vi "Initialize.vi"(8 "error in":errorcluster, 11 "Plugin in":refnum<class "Tone Measurements.lvclass">) -> (0 "error out":errorcluster, 3 "Plugin out":refnum<class "Tone Measurements.lvclass">)   [LabVIEW 2025, in "Tone Measurements.lvlib" / "Tone Measurements.lvclass"]
uses:
  Tone Measurements.lvclass
  C:/Program Files/National Instruments/LabVIEW 2025/vi.lib/FlexLogger/SDK/PluginSDK.lvlibp/PEFClasses/SDK/Plugin/Plugin.lvclass
  <vilib>/FlexLogger/SDK/PluginSDK.lvlibp/PEFClasses/SDK/Producer Channel/Producer Channel.lvclass
  C:/Program Files/National Instruments/LabVIEW 2025/vi.lib/FlexLogger/SDK/PluginSDK.lvlibp/PEFClasses/SDK/Channel/Channel.lvclass
  <vilib>/FlexLogger/SDK/PluginSDK.lvlibp/PEFClasses/SDK/Plugin/ParameterAccess/Write Single Channel.vi
  <vilib>/FlexLogger/SDK/PluginSDK.lvlibp/PEFClasses/SDK/Plugin/ParameterAccess/Write DBL.vi
  <vilib>/FlexLogger/SDK/PluginSDK.lvlibp/PEFClasses/SDK/Plugin/ParameterAccess/Write I32.vi
  <vilib>/FlexLogger/SDK/PluginSDK.lvlibp/PEFClasses/SDK/Producer Channel/Create Producer Channel_v2.vi
  <vilib>/FlexLogger/SDK/PluginSDK.lvlibp/PEFClasses/SDK/Plugin/Plugin.lvclass
  C:/Program Files/National Instruments/LabVIEW 2025/vi.lib/FlexLogger/SDK/PluginSDK.lvlibp/PEFClasses/SDK/Processing Element/Processing Element.lvclass
  C:/dev/dsb/niflexlogger-plugins/PDK plugins/Tone Measurements/Tone Measurements.lvclass
  <vilib>/FlexLogger/SDK/PluginSDK.lvlibp
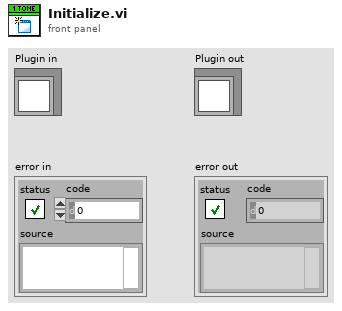
[diagram p1: front panel]
types:
  T1 = cluster{"Unique Channel Identifier":string, "Long Name":string, "Unit":string}[]
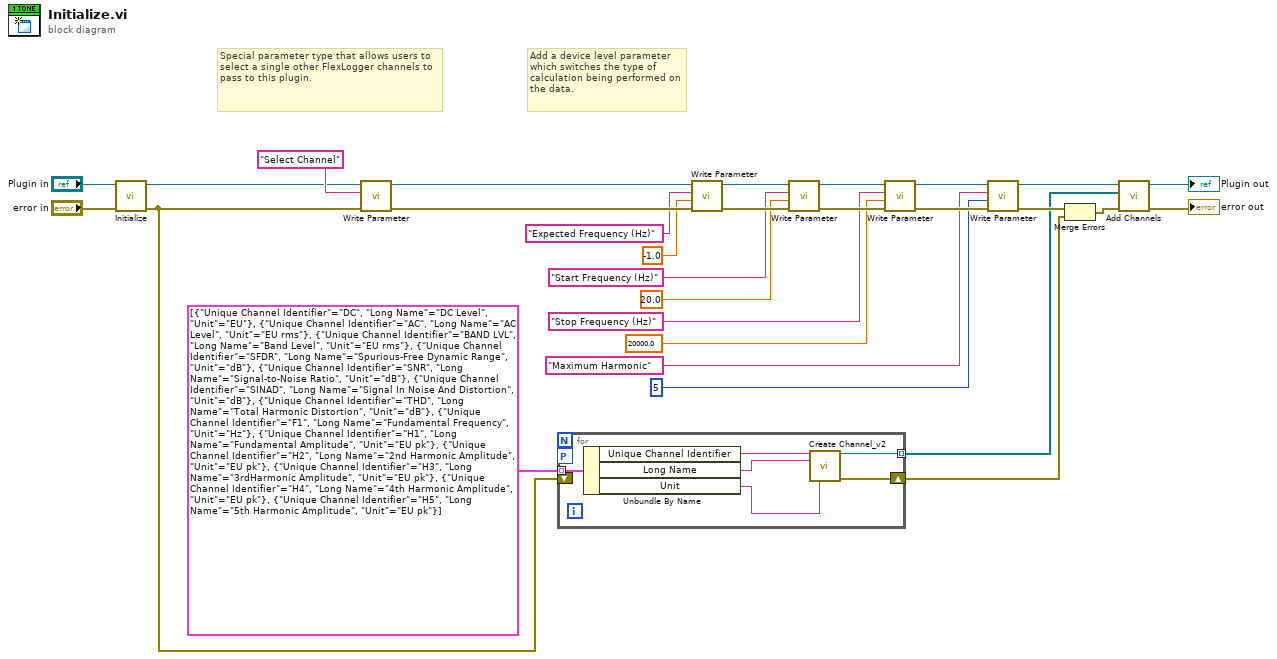
[diagram p0: block diagram]
diagram:
  # "Add a device level parameter which switches the type of calculation being performed on the data."
  # "Special parameter type that allows users to select a single other FlexLogger channels to pass to this plugin."
  n1 = call-parent "Initialize.vi"("error in (no error)"="error in", "Plugin in"="Plugin in") -> ("error out"=w2:errorcluster, "Plugin out"=w21:refnum<class "Tone Measurements.lvclass">)  [unwired: 8 in]
  n2 = call-poly <vilib>:"Write Parameter.vi"("error in (no error)"=w2, "Name (Unique Channel Identifier)"="Select Channel" ("Name"), "Plugin in"=w21) -> ("error out"=w23:errorcluster, "Plugin out"=w24:refnum<class "Tone Measurements.lvclass">)  [unwired: 7 in]
  n3 = for {
    tunnel: T1 [{"Unique Channel Identifier"="DC", "Long Name"="DC Level", "Unit"="EU"}, {"Unique Channel Identifier"="AC", "Long Name"="AC Level", "Unit"="EU rms"}, {"Unique Channel Identifier"="BAND LVL", "Long Name"="Band Level", "Unit"="EU rms"}, {"Unique Channel Identifier"="SFDR", "Long Name"="Spurious-Free Dynamic Range", "Unit"="dB"}, {"Unique Channel Identifier"="SNR", "Long Name"="Signal-to-Noise Ratio", "Unit"="dB"}, {"Unique Channel Identifier"="SINAD", "Long Name"="Signal In Noise And Distortion", "Unit"="dB"}, {"Unique Channel Identifier"="THD", "Long Name"="Total Harmonic Distortion", "Unit"="dB"}, {"Unique Channel Identifier"="F1", "Long Name"="Fundamental Frequency", "Unit"="Hz"}, {"Unique Channel Identifier"="H1", "Long Name"="Fundamental Amplitude", "Unit"="EU pk"}, {"Unique Channel Identifier"="H2", "Long Name"="2nd Harmonic Amplitude", "Unit"="EU pk"}, {"Unique Channel Identifier"="H3", "Long Name"="3rdHarmonic Amplitude", "Unit"="EU pk"}, {"Unique Channel Identifier"="H4", "Long Name"="4th Harmonic Amplitude", "Unit"="EU pk"}, {"Unique Channel Identifier"="H5", "Long Name"="5th Harmonic Amplitude", "Unit"="EU pk"}] -> [w35] mode=indexing
    tunnel: [w31] -> w3 mode=indexing
    workers-P: _ -> [_]
    shift-right: [w30] -> w1
    shift-left: w2 -> [_]
    n4 = Unbundle By Name(w35) -> ("Unique Channel Identifier"=w34:string, "Long Name"=w33:string, "Unit"=w32:string)
    n5 = call-poly <vilib>:"Create Channel_v2.vi"("Unique Channel Identifier"=w34, "Default Channel Name"=w33, "Unit"=w32) -> ("Producer Channel"=w31:refnum<class "Producer Channel.lvclass">, "error out"=w30:errorcluster)  [unwired: 11 in]
  }
  n6 = call-poly <vilib>:"Write Parameter.vi"("error in (no error)"=w23, "Value"=-1.0, "Name"="Expected Frequency (Hz)", "Plugin in"=w24) -> ("error out"=w18:errorcluster, "Plugin out"=w19:refnum<class "Tone Measurements.lvclass">)  [unwired: 6 in]
  n7 = call-poly <vilib>:"Write Parameter.vi"("error in (no error)"=w18, "Value"=20.0, "Name"="Start Frequency (Hz)", "Plugin in"=w19) -> ("error out"=w17:errorcluster, "Plugin out"=w16:refnum<class "Tone Measurements.lvclass">)  [unwired: 6 in]
  n8 = call-poly <vilib>:"Write Parameter.vi"("error in (no error)"=w17, "Value"=20000.0, "Name"="Stop Frequency (Hz)", "Plugin in"=w16) -> ("error out"=w15:errorcluster, "Plugin out"=w14:refnum<class "Tone Measurements.lvclass">)  [unwired: 6 in]
  n9 = call-poly <vilib>:"Write Parameter.vi"("error in (no error)"=w15, "Value"=5, "Name"="Maximum Harmonic", "Plugin in"=w14) -> ("error out"=w6:errorcluster, "Plugin out"=w13:refnum<class "Tone Measurements.lvclass">)  [unwired: 6 in]
  n10 = Merge Errors(w6, w1) -> (w5:errorcluster)
  n11 = call <vilib>:"Add Channels.vi"("error in (no error)"=w5, "Channels"=w3, "Plugin in"=w13) -> ("error out"=→"error out":errorcluster, "Plugin out"=→"Plugin out":refnum<class "Tone Measurements.lvclass">)  [unwired: 7 in]
